vi "(SubVI) Pull DNA_ver2PI_YCC.vi"(1 "Filter type":T1(ring), 2 "Avg points":i32, 5 "Record?":bool, 7 "T=X\nF=Y":bool, 9 "Toward  ?\nT=+, F=-":bool, 11 "no Record scan rate  (um/s)":dbl=2.0, 12 "Record scan rate  (um/s)":dbl=2.0 format="%.3f", 13 "range  (um)":dbl=2.0 min=0.0 max=100.0 step=0.5 format="%.3f", 14 "Sampling rate":dbl=20000.0 format="%0.2f") -> (6 "Raw Stage Array":dbl[](array[numeric]), 8 "Filtered Stage Array":dbl[](array[numeric]) format="%0.2f", 10 "Filtered QPD Array":dbl[](array[numeric]) format="%0.2f")   [LabVIEW 2014]
panel:
  out "Start From  (um)":dbl min=0.0 max=100.0 step=0.5 format="%.3f"
  out "delay (ms)":dbl
  out "scan rate  (um/s)":dbl
  out "axis":u32=1
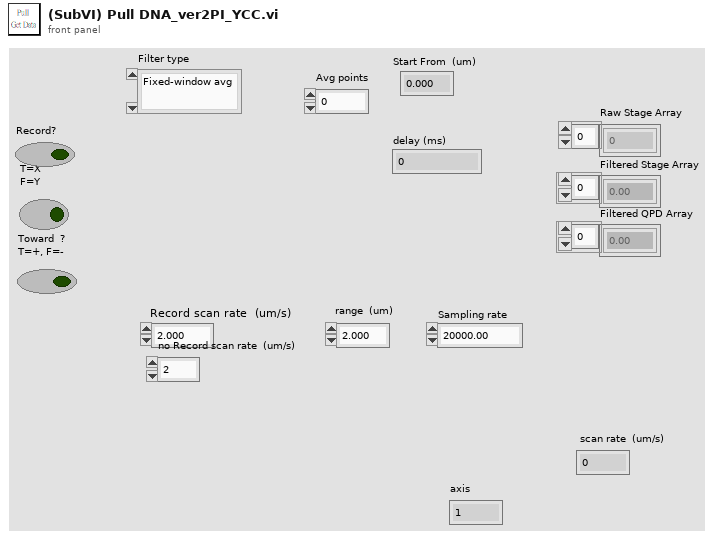
[diagram p1: front panel]
types:
  T1 = enum16{"Fixed-window avg", "Moving-window avg", "F+S-window avg", "S-G filter", "Fixed-window Median", "Moving-window Median "}
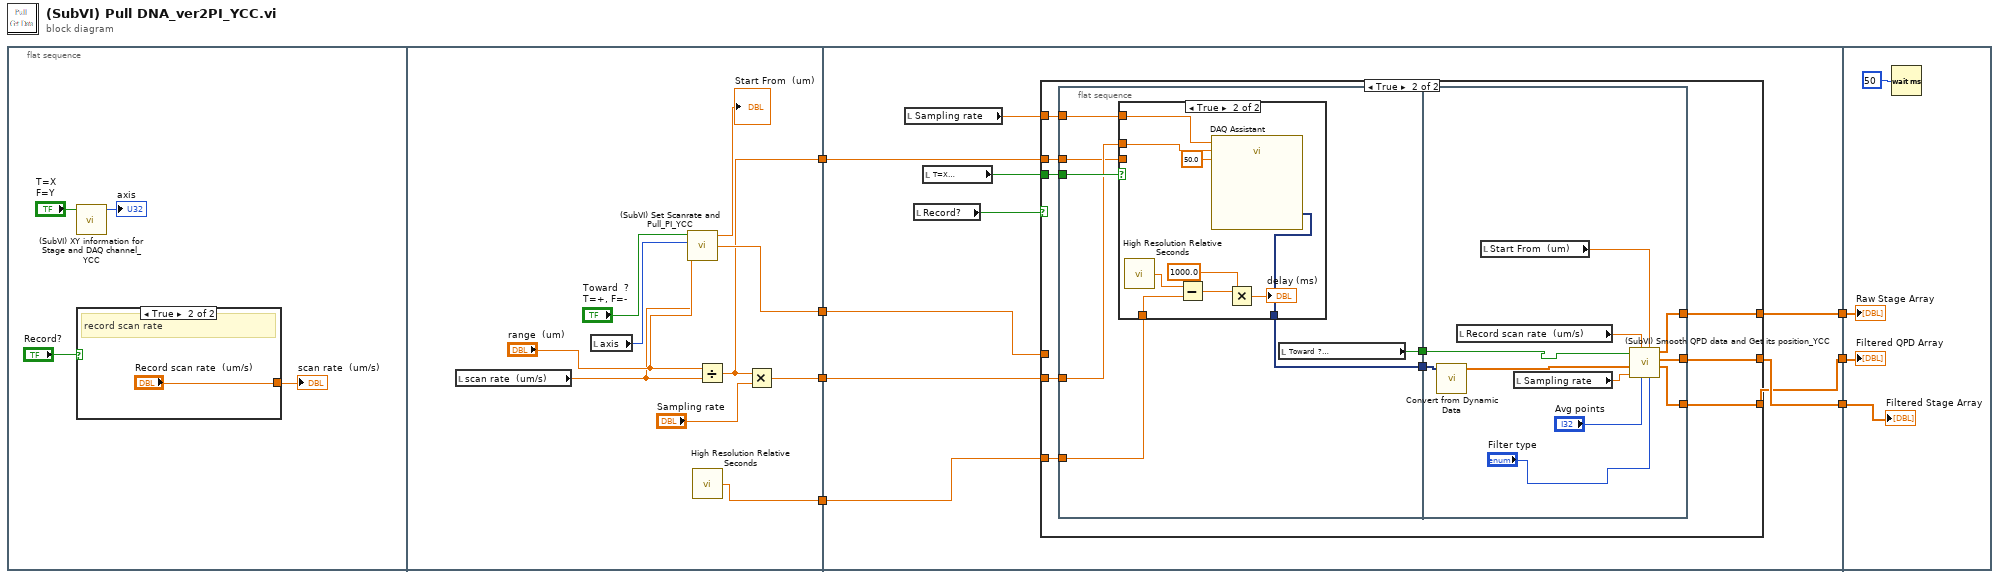
[diagram p0: block diagram]
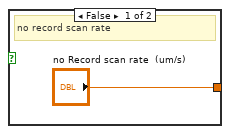
[diagram p2: hidden frame]
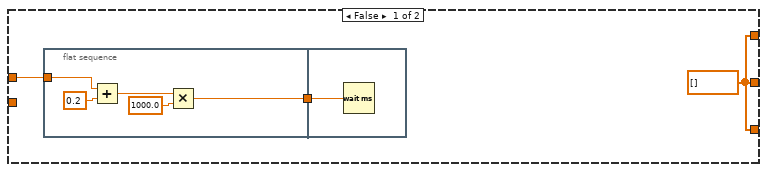
[diagram p3: hidden frame]
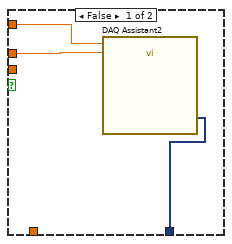
[diagram p4: hidden frame]
diagram:
  n1 = flat-sequence {
    tunnel: [w22] -> w4
    tunnel: [w17] -> w3
    tunnel: [w16] -> w2
    tunnel: [w15] -> w1
    tunnel: [w31] -> w7
    tunnel: [w30] -> w6
    tunnel: [w29] -> w5
    tunnel: w2 -> [w25]
    tunnel: w3 -> [w26]
    tunnel: w4 -> [w33]
    tunnel: w1 -> [w24]
    tunnel: w7 -> [w86]
    tunnel: w6 -> [w85]
    tunnel: w5 -> [w84]
    frame #0 {
      n2 = call "(SubVI) XY information for Stage and DAQ channel_YCC.vi"("T=X\nF=Y"="T=X\nF=Y") -> ("Axis"=→"axis":i32)  [unwired: 3 in, 1 out]
      n3 = case shown="True" "Record?" {
        tunnel: ["no Record scan rate  (um/s)" "Record scan rate  (um/s)"] -> w8
        frame False {
          # "no record scan rate"
        }
        frame True {
          # "record scan rate"
        }
      }
      "scan rate  (um/s)" <- w8
    }
    frame #1 {
      n4 = local read "scan rate  (um/s)"() -> (w18:dbl)
      n5 = local read "axis"() -> (w23:u32)
      n6 = call "(SubVI) Set Scanrate and Pull_PI_YCC.vi"("toward+ ?\nT=+, F=-"="Toward  ?\nT=+, F=-", "axis"=w23, "scan rate  (um/s)"=w18, "range  (um)"="range  (um)") -> ("Start From  (um)"=→"Start From  (um)":dbl, "Traveling time (s)"=w17:dbl)  [unwired: 3 in]
      n7 = call <vilib>:"High Resolution Relative Seconds.vi"() -> ("relative seconds"=w15:dbl)
      n8 = Divide(x="range  (um)", y=w18) -> (x/y=w16:dbl)
      n9 = Multiply(x=w16, y="Sampling rate") -> (x*y=w22:dbl)
    }
    frame #2 {
      n10 = local read "Sampling rate"() -> (w27:dbl)
      n11 = local read "Record?"() -> (w32:bool)
      n12 = local read "T=X\nF=Y"() -> (w28:bool)
      n13 = case shown="True" w32 {
        tunnel: w33 -> [_ w52]
        tunnel: [w36 w49] -> w31
        tunnel: [w36 w48] -> w29
        tunnel: [w36 w47] -> w30
        tunnel: w28 -> [_ w46]
        tunnel: w27 -> [_ w45]
        tunnel: w26 -> [w34 _]
        tunnel: w25 -> [_ w44]
        tunnel: w24 -> [_ w43]
        frame False {
          w36 = dbl[] [] ("data")
          n14 = flat-sequence {
            tunnel: [w40] -> w35
            tunnel: w34 -> [w37]
            tunnel: w35 -> [w42]
            frame #0 {
              n15 = Add(x=w37, y=0.2) -> (x+y=w38:dbl)
              n16 = Multiply(x=w38, y=1000.0) -> (x*y=w40:dbl)
            }
            frame #1 {
              n17 = Wait (ms)(milliseconds to wait=w42) -> ()  [unwired: 1 out]
            }
          }
        }
        frame True {
          n18 = flat-sequence {
            tunnel: w52 -> [w55]
            tunnel: [w59] -> w51
            tunnel: [w56] -> w50
            tunnel: w46 -> [w58]
            tunnel: w45 -> [w57]
            tunnel: w44 -> [w54]
            tunnel: w43 -> [w53]
            tunnel: w51 -> [w74]
            tunnel: w50 -> [w78]
            tunnel: [w77] -> w49
            tunnel: [w76] -> w48
            tunnel: [w75] -> w47
            frame #0 {
              n19 = case shown="True" w58 {
                tunnel: w57 -> [w62 w71]
                tunnel: [w61 w69] -> w56
                tunnel: w55 -> [w60 w70]
                tunnel: w54 -> [_ _]
                tunnel: w53 -> [_ w64]
                frame False {
                  n20 = call "DAQ Assistant2"("rate"=w62, "number of samples"=w60) -> ("data"=w61:dynamicdata)  [unwired: 15 in, 2 out]
                }
                frame True {
                  n21 = call <vilib>:"High Resolution Relative Seconds.vi"() -> ("relative seconds"=w68:dbl)
                  n22 = Subtract(x=w68, y=w64) -> (x-y=w67:dbl)
                  n23 = call "DAQ Assistant"("rate"=w71, "number of samples"=w70, "timeout (s)"=50.0) -> ("data"=w69:dynamicdata)  [unwired: 14 in, 2 out]
                  n24 = Multiply(x=w67, y=1000.0) -> (x*y=→"delay (ms)":dbl)
                }
              }
              n25 = local read "Toward  ?\nT=+, F=-"() -> (w59:bool)
            }
            frame #1 {
              n26 = call "Convert from Dynamic Data"("Dynamic Data Type"=w78) -> ("Array"=w73:dbl[])  [unwired: 3 in]
              n27 = local read "Record scan rate  (um/s)"() -> (w79:dbl)
              n28 = local read "Start From  (um)"() -> (w82:dbl)
              n29 = local read "Sampling rate"() -> (w81:dbl)
              n30 = call "(SubVI) Smooth QPD data and Get its position_YCC.vi"("Filter type"="Filter type", "Initial position (um)"=w82, "Avg points"="Avg points", "scan rate  (um/s)"=w79, "Sampling rate (Hz)"=w81, "QPD data"=w73, "Direction\nT=+ \nF=-"=w74) -> ("Filtered QPD data"=w76:dbl[], "Filtered Stage Array"=w75:dbl[], "Raw Stage Array"=w77:dbl[])  [unwired: 2 in]
            }
          }
        }
      }
    }
    frame #3 {
      n31 = Wait (ms)(milliseconds to wait=u32 50) -> ()  [unwired: 1 out]
      "Raw Stage Array" <- w86
      "Filtered Stage Array" <- w85
      "Filtered QPD Array" <- w84
    }
  }
